vi "UpdateShotPositions.vi"(1 "Direction":T1, 2 "ShotPos_IN":T2(array[cluster]), 3 "Speed":i16) -> (0 "ShotPos_OUT":T2(array[cluster]))   [LabVIEW 2019]
uses:
  shot_direction.ctl
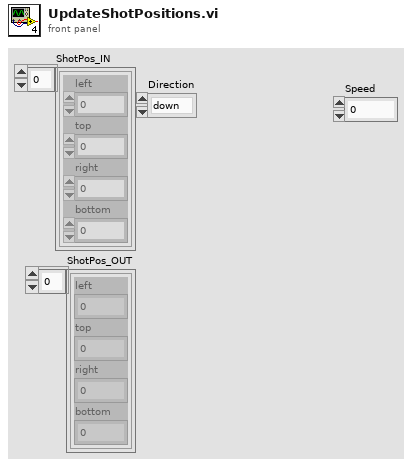
[diagram p1: front panel]
types:
  T1 = typedef "shot_direction.ctl" = enum16{"down", "up"}
  T2 = cluster{"left":i16, "top":i16, "right":i16, "bottom":i16}[]
  T3 = cluster{"left":i16, "top":i16, "right":i16, "bottom":i16}
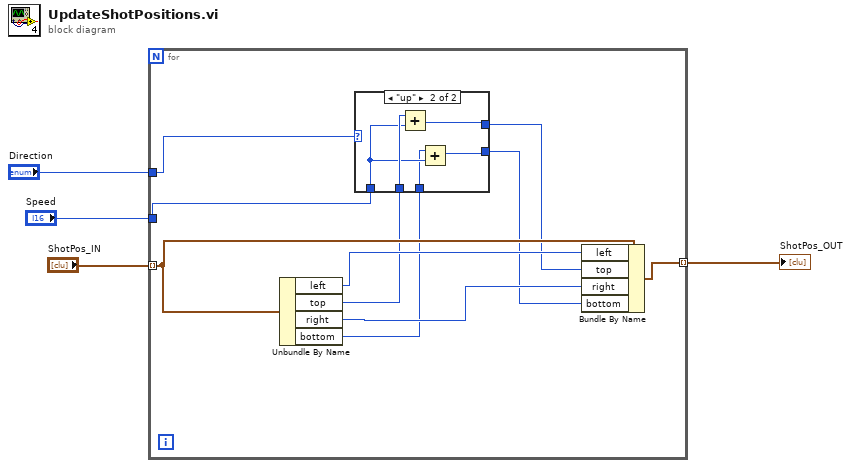
[diagram p0: block diagram]
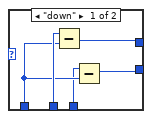
[diagram p2: hidden frame]
diagram:
  n1 = for {
    tunnel: "ShotPos_IN" -> [w14] mode=indexing
    tunnel: [w11] -> w3 mode=indexing
    tunnel: "Speed" -> [w9]
    tunnel: "Direction" -> [w10]
    n2 = Unbundle By Name(w14) -> ("left"=w13:i16, "top"=w8:i16, "right"=w12:i16, "bottom"=w6:i16)
    n3 = case shown="\"up\"" w10 {
      tunnel: w9 -> [w17 w22]
      tunnel: w8 -> [w19 w24]
      tunnel: [w18 w23] -> w7
      tunnel: w6 -> [w16 w21]
      tunnel: [w15 w20] -> w5
      frame "down" {
        n4 = Subtract(x=w19, y=w17) -> (x-y=w18:i16)
        n5 = Subtract(x=w16, y=w17) -> (x-y=w15:i16)
      }
      frame "up" {
        n6 = Add(x=w24, y=w22) -> (x+y=w23:i16)
        n7 = Add(x=w21, y=w22) -> (x+y=w20:i16)
      }
    }
    n8 = Bundle By Name(cluster=w14, "left"=w13, "top"=w7, "right"=w12, "bottom"=w5) -> (w11:T3)
  }
  "ShotPos_OUT" <- w3
